vi "取范围.vi"(8 "max":dbl, 9 "min":dbl, 10 "y":dbl[](array[numeric]), 11 "x":dbl[](array[numeric])) -> (2 "y":dbl[](array[numeric]), 3 "x":dbl[](array[numeric]))   [LabVIEW 2015]
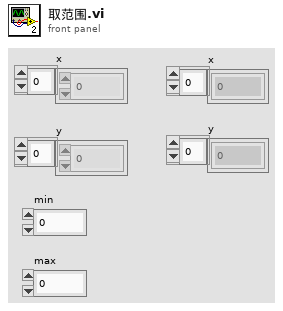
[diagram p1: front panel]
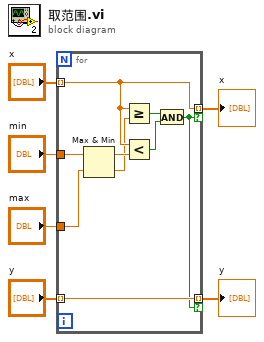
[diagram p0: block diagram]
diagram:
  n1 = for {
    tunnel: "x" -> [w13] mode=indexing
    tunnel: [w13] -> w3 mode=indexing if=w11
    tunnel: "y" -> [w12] mode=indexing
    tunnel: [w12] -> w4 mode=indexing if=w11
    tunnel: "min" -> [w10]
    tunnel: "max" -> [w9]
    n2 = Max & Min(x=w10, y=w9) -> (max(x,y)=w8:dbl, min(x,y)=w7:dbl)
    n3 = Greater Or Equal?(x=w13, y=w7) -> (x >= y?=w15:bool)
    n4 = Less?(x=w13, y=w8) -> (x < y?=w14:bool)
    n5 = And(x=w15, y=w14) -> (x .and. y?=w11:bool)
  }
  "y" <- w4
  "x" <- w3
